vi "Loader.vi"(8 "error in (no error)":errorcluster, 10 "Path":path, 11 "Config_Read_SPI.lvclass":refnum<class "Config_Read_SPI.lvclass">) -> (0 "error out":errorcluster, 1 "Pattern_Name":string, 2 "SPI_FRM_Array":T1[](array[typedef]) {"Addr" format="%x"; "Data" format="%x"}, 3 "Config_Read_SPI.lvclass out":refnum<class "Config_Read_SPI.lvclass">)   [LabVIEW 2018, in "Config_Read_SPI.lvclass"]
uses:
  Config_Read_SPI.lvclass
  SPI_FRM_Config.ctl
  Classes/Config_Read/RW_Option.ctl
  SPI_Mode.ctl
  Config_Read_SPI.lvclass/Config_Read_SPI.ctl
  Classes/Config_Read/Config_Read_BML.lvclass
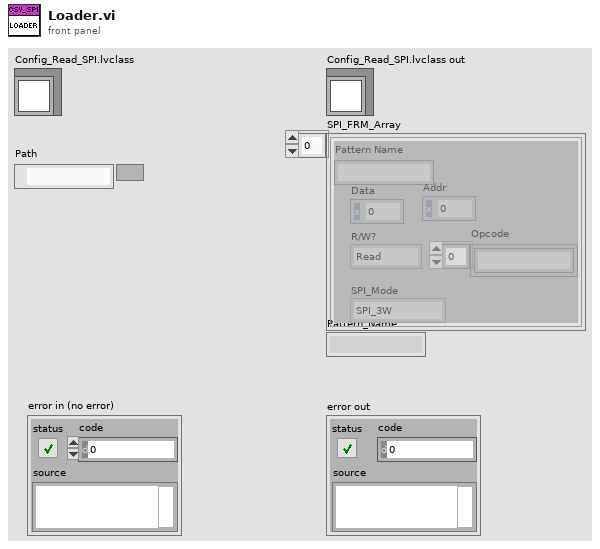
[diagram p1: front panel]
types:
  T1 = typedef "Config_Read_SPI.lvclass/SPI_FRM_Config.ctl" = cluster{"Pattern Name":string, "Data":u16, "Addr":u16, "R/W?":T2, "Opcode":string[], "SPI_Mode":T3}
  T2 = typedef "Config_Read_BML.lvclass/RW_Option.ctl" = enum16{"Read", "Write", "R/W"}
  T3 = typedef "Config_Read_SPI.lvclass/SPI_Mode.ctl" = enum16{"SPI_3W", "SPI_4W"}
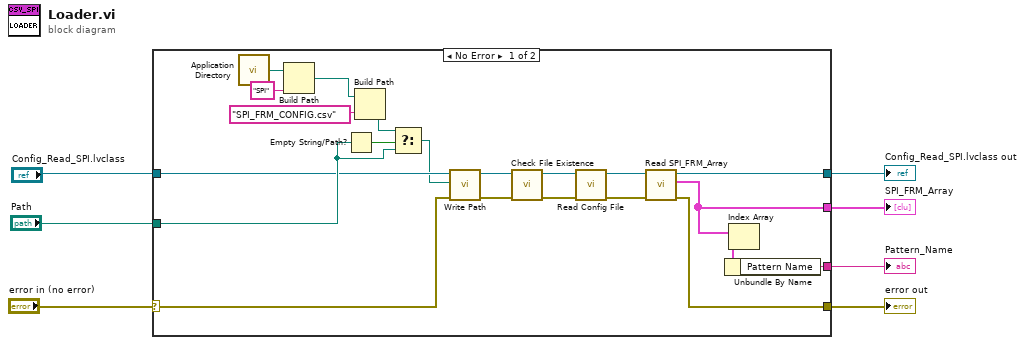
[diagram p0: block diagram]
diagram:
  n1 = case shown="No Error" "error in (no error)" {
    selector: "error in (no error)" -> [w22 w30]
    tunnel: "Config_Read_SPI.lvclass" -> [w23 w29]
    tunnel: "Path" -> [w27 _]
    tunnel: [w14 w29] -> w1
    tunnel: [w12 w30] -> w5
    tunnel: [w24 _] -> w3
    tunnel: [w11 _] -> w2
    frame No Error {
      n2 = call <vilib>:"Application Directory.vi"() -> ("Application Directory"=w10:path)
      n3 = Build Path(base path=w10, name or relative path="SPI") -> (appended path=w8:path)
      n4 = Empty String/Path?(string/path=w27) -> (empty?=w28:bool)
      n5 = Build Path(base path=w8, name or relative path="SPI_FRM_CONFIG.csv") -> (appended path=w25:path)
      n6 = Select(t=w25, s=w28, f=w27) -> (s? t:f=w21:path)
      n7 = call "Write Path.vi"("error in (no error)"=w22, "Path"=w21, "Config_Read_SPI in"=w23) -> ("error out"=w19:errorcluster, "Config_Read_SPI out"=w20:refnum<class "Config_Read_SPI.lvclass">)  [unwired: 7 in]
      n8 = call "Check File Existence.vi"("error in (no error)"=w19, "Config_Read_SPI.lvclass"=w20) -> ("error out"=w17:errorcluster, "Config_Read_SPI.lvclass out"=w18:refnum<class "Config_Read_SPI.lvclass">)  [unwired: 8 in]
      n9 = call "Read Config File.vi"("error in (no error)"=w17, "Config_Read_SPI.lvclass"=w18) -> ("error out"=w15:errorcluster, "Config_Read_SPI.lvclass out"=w16:refnum<class "Config_Read_SPI.lvclass">)  [unwired: 8 in]
      n10 = call "Read SPI_FRM_Array.vi"("error in (no error)"=w15, "Config_Read_SPI in"=w16) -> ("error out"=w12:errorcluster, "SPI_FRM_Array"=w11:T1[], "Config_Read_SPI out"=w14:refnum<class "Config_Read_SPI.lvclass">)  [unwired: 7 in]
      n11 = Index Array(array=w11) -> (element=w13:T1)  [unwired: 1 in]
      n12 = Unbundle By Name(w13) -> ("Pattern Name"=w24:string)
    }
    frame Error {
    }
  }
  "error out" <- w5
  "Pattern_Name" <- w3
  "SPI_FRM_Array" <- w2
  "Config_Read_SPI.lvclass out" <- w1
